vi "QMH_handError_Notifier.vi"(8 "error in (no error)":errorcluster) -> (0 "error out":errorcluster)   [LabVIEW 2021, in "Framework_lib.lvlib"]
uses:
  Framework_lib.lvlib
  QMH_producer_enum.ctl
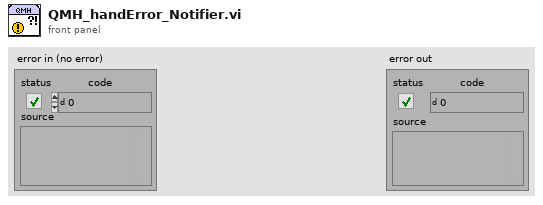
[diagram p1: front panel]
types:
  T1 = typedef "Framework_lib.lvlib/QMH_producer_enum.ctl" = enum16{"Idle", "Initialize", "Shutdown", "ERROR", "Stop", "Start", "Enqueue_frames", "Paused", "Resume"}
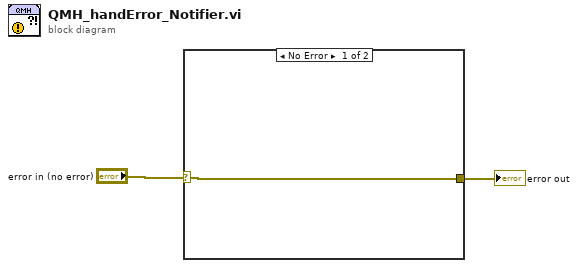
[diagram p0: block diagram]
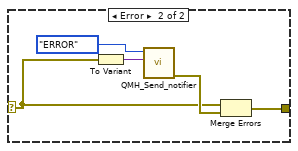
[diagram p2: hidden frame]
diagram:
  n1 = case shown="No Error" "error in (no error)" {
    selector: "error in (no error)" -> [w3 w4]
    tunnel: [w3 w5] -> w1
    frame No Error {
    }
    frame Error {
      n2 = To Variant(anything=w4) -> (Variant=w7:variant)
      n3 = call "QMH_Send_notifier.vi"("Payload"=w7, "Message"=QMH_producer_enum."ERROR") -> ("error out"=w8:errorcluster)  [unwired: 9 in]
      n4 = Merge Errors(w4, w8) -> (w5:errorcluster)
    }
  }
  "error out" <- w1
